vi "aes_VVT Offset Angle.vi"(6 "Using Cycle Angle":bool, 9 "Cam.Offset":fxp<+/-,61,10>, 11 "Crank or Cyle Angle":fxp<+,61,10>) -> (3 "Crank.Adjusted Offset Angle":fxp<+,61,10> format="%.55g")   [LabVIEW 2010, in "AES.lvlib" / "AES FPGA.lvlib"]
doc: "This IP applies an adjustable offset to the crank angle that will offset the time that our Cam output is updated. Essentially this IP offsets the cam angles stored in memory of the Cam Angle and Output VVT.vi to provide VVT functionality for the Cam."
uses:
  AES FPGA.lvlib
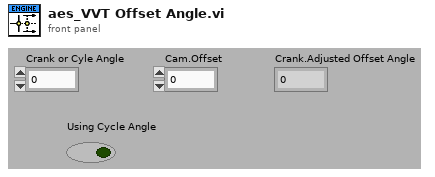
[diagram p1: front panel]
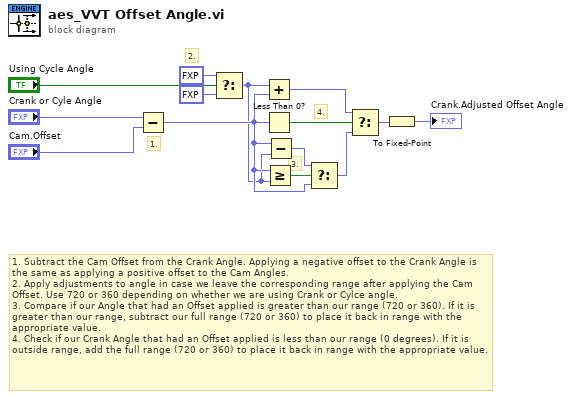
[diagram p0: block diagram]
diagram:
  # "1. Subtract the Cam Offset from the Crank Angle. Applying a negative offset to the Crank Angle is the same as applying a positive offset to the Cam Angles.\n2. Apply adjustments to angle in case we leave the corresponding range after applying the Cam Offset. Use 720 or 360 depending on whether we are using Crank or Cylce angle.\n3. Compare if our Angle that had an Offset applied is greater than our range (720 or 360). If it is greater than our range, subtract our full range (720 or 360) to place it back in range with the appropriate value.\n4. Check if our Crank Angle that had an Offset applied is less than our range (0 degrees). If it is outside range, add the full range (720 or 360) to place it back in range with the appropriate value."
  # "4."
  # "3."
  # "2."
  # "1."
  n1 = Subtract(x="Crank or Cyle Angle", y="Cam.Offset") -> (x-y=w9:fxp<+/-,63,12>)
  n2 = Select(t=fxp<+,7,10> 720.0 ("x"), s="Using Cycle Angle", f=fxp<+,6,9> 360.0 ("x")) -> (s? t:f=w3:fxp<+,7,10>)
  n3 = Add(x=w3, y=w9) -> (x+y=w12:fxp<+/-,64,13>)
  n4 = Less Than 0?(x=w9) -> (x < 0?=w13:bool)
  n5 = Greater Or Equal?(x=w9, y=w3) -> (x >= y?=w11:bool)
  n6 = Subtract(x=w9, y=w3) -> (x-y=w10:fxp<+/-,63,12>)
  n7 = Select(t=w10, s=w11, f=w9) -> (s? t:f=w8:fxp<+/-,63,12>)
  n8 = Select(t=w12, s=w13, f=w8) -> (s? t:f=w6:fxp<+/-,64,13>)
  n9 = To Fixed-Point(number=w6) -> (fixed-point=→"Crank.Adjusted Offset Angle":fxp<+,61,10>)  [unwired: 1 in]
